vi "FTW-Message-Multipart-Interpret.vi"(0 "FTW Message":refnum<class "FTW-Message-Lossy.lvclass">, 11 "error in":errorcluster) -> (4 "FTW Message out":refnum<class "FTW-Message-Lossy.lvclass">, 6 "Message Parts":string[](array[string]), 15 "error out":errorcluster)   [LabVIEW 2013]
uses:
  FTW-Message-Lossy.lvclass
panel:
  # "Inputs"
  # "Outputs"
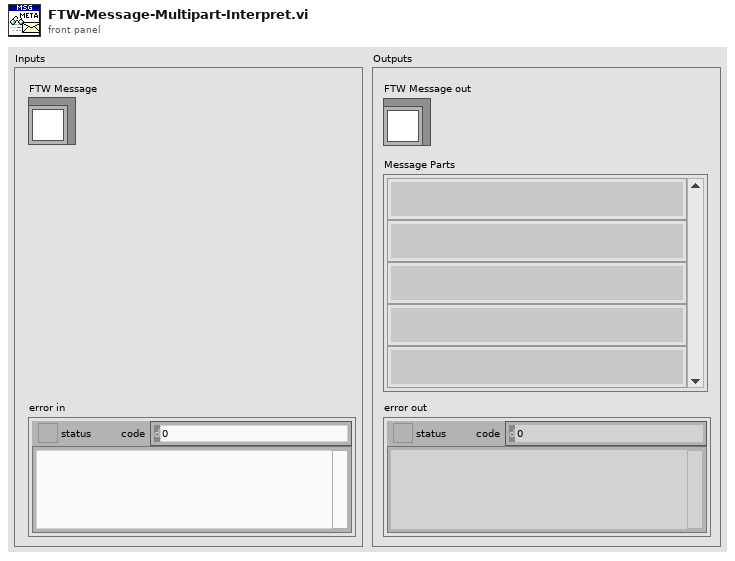
[diagram p1: front panel]
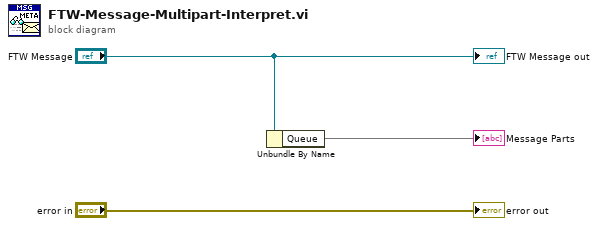
[diagram p0: block diagram]
diagram:
  n1 = Unbundle By Name("FTW Message") -> ("Queue"=→"Message Parts")
  "error out" <- "error in"
  "FTW Message out" <- "FTW Message"
